vi "Start Wfms.vi"(8 "error in (no error)":errorcluster, 11 "Compiled.Settings":T2={"Name"="", "Async Init Timeout"=0, "File Data"={"Date Captured"="", "Directory"="", "Name"="", "Groups"=[], "Meta Data"=[]}, "Segment Files"=FALSE, "Segment Every"=0.0, "Trigger?"=FALSE, "Segment by"=enum."Size (MB)", "Trigger Ref"=0} {"Trigger Ref" format="%.0x"; "File Data"."Groups"."Channels"."Data Reference in" format="%.0x"}) -> (0 "error out":errorcluster, 1 "Channel Refs":T1[](array[typedef]) format="%.0x", 2 "Wfm Refs":refnum<class "Single Waveform Read (DBL).lvclass">[](array[class]), 3 "Compiled.Settings Out":T2={"Name"="", "Async Init Timeout"=0, "File Data"={"Date Captured"="", "Directory"="", "Name"="", "Groups"=[], "Meta Data"=[]}, "Segment Files"=FALSE, "Segment Every"=0.0, "Trigger?"=FALSE, "Segment by"=enum."Size (MB)", "Trigger Ref"=0} {"Trigger Ref" format="%.0x"; "File Data"."Groups"."Channels"."Data Reference in" format="%.0x"})   [LabVIEW 2023, in "Embedded TDMS Logger Engine.lvlib"]
uses:
  Embedded TDMS Logger Engine.lvlib
  Shared/Compiled.Settings.ctl
  Shared/FileData.ctl
  Shared/GroupData.ctl
  Shared/Meta Data Item.ctl
  Shared/ChannelData.ctl
  <vilib>/NI VeriStand/Custom Device API/Data Reference.ctl
  Shared/SegmentOptions.ctl
  <vilib>/NI VeriStand/Custom Device Waveform API/Single Waveform Read (DBL)/Single Waveform Read (DBL).lvclass
  <vilib>/NI VeriStand/Custom Device Waveform API/Single Waveform Read (DBL)/NI VeriStand - Open Single Waveform Read Session (DBL).vi
  <vilib>/NI VeriStand/Custom Device Waveform API/NI_VS Custom Device Waveform API.lvlib
  Shared/Embedded TDMS Logger Shared.lvlib
  <vilib>/NI VeriStand/Custom Device API/Custom Device API.lvlib
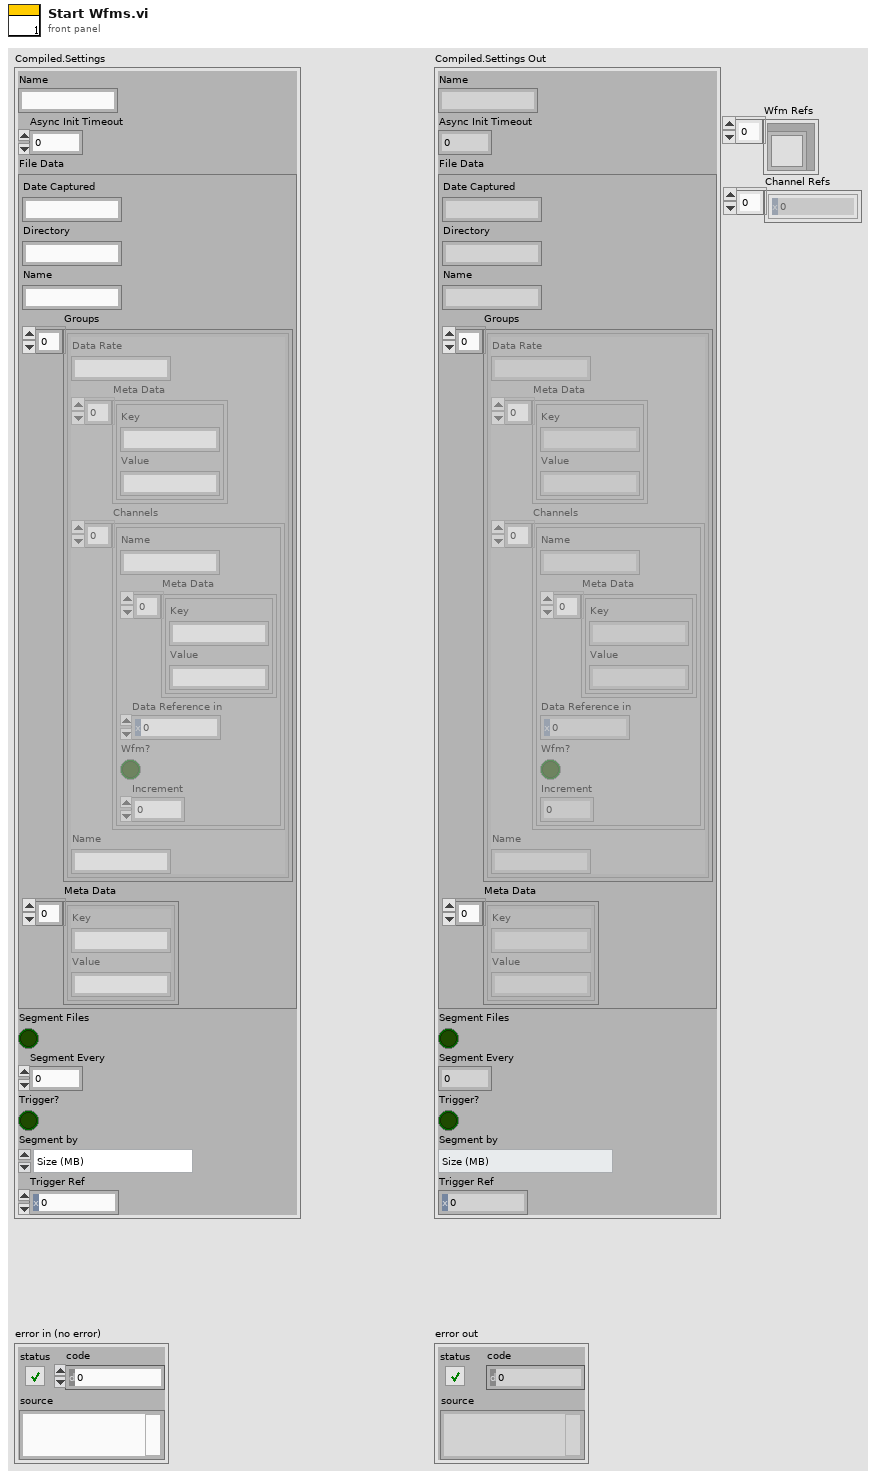
[diagram p1: front panel]
types:
  T1 = typedef "Custom Device API.lvlib/Data Reference.ctl" = i32
  T2 = typedef "Embedded TDMS Logger Shared.lvlib/Compiled.Settings.ctl" = cluster{"Name":string, "Async Init Timeout":u16, "File Data":T3, "Segment Files":bool, "Segment Every":dbl, "Trigger?":bool, "Segment by":T7, "Trigger Ref":T1}
  T3 = typedef "Embedded TDMS Logger Shared.lvlib/FileData.ctl" = cluster{"Date Captured":string, "Directory":string, "Name":string, "Groups":T4[], "Meta Data":T5[]}
  T4 = typedef "Embedded TDMS Logger Shared.lvlib/GroupData.ctl" = cluster{"Data Rate":string, "Meta Data":T5[], "Channels":T6[], "Name":string}
  T5 = typedef "Embedded TDMS Logger Shared.lvlib/Meta Data Item.ctl" = cluster{"Key":string, "Value":string}
  T6 = typedef "Embedded TDMS Logger Shared.lvlib/ChannelData.ctl" = cluster{"Name":string, "Meta Data":T5[], "Data Reference":T1, "Wfm?":bool, "Increment":dbl}
  T7 = typedef "SegmentOptions.ctl" = enum16{"Time (s)", "Size (MB)"}
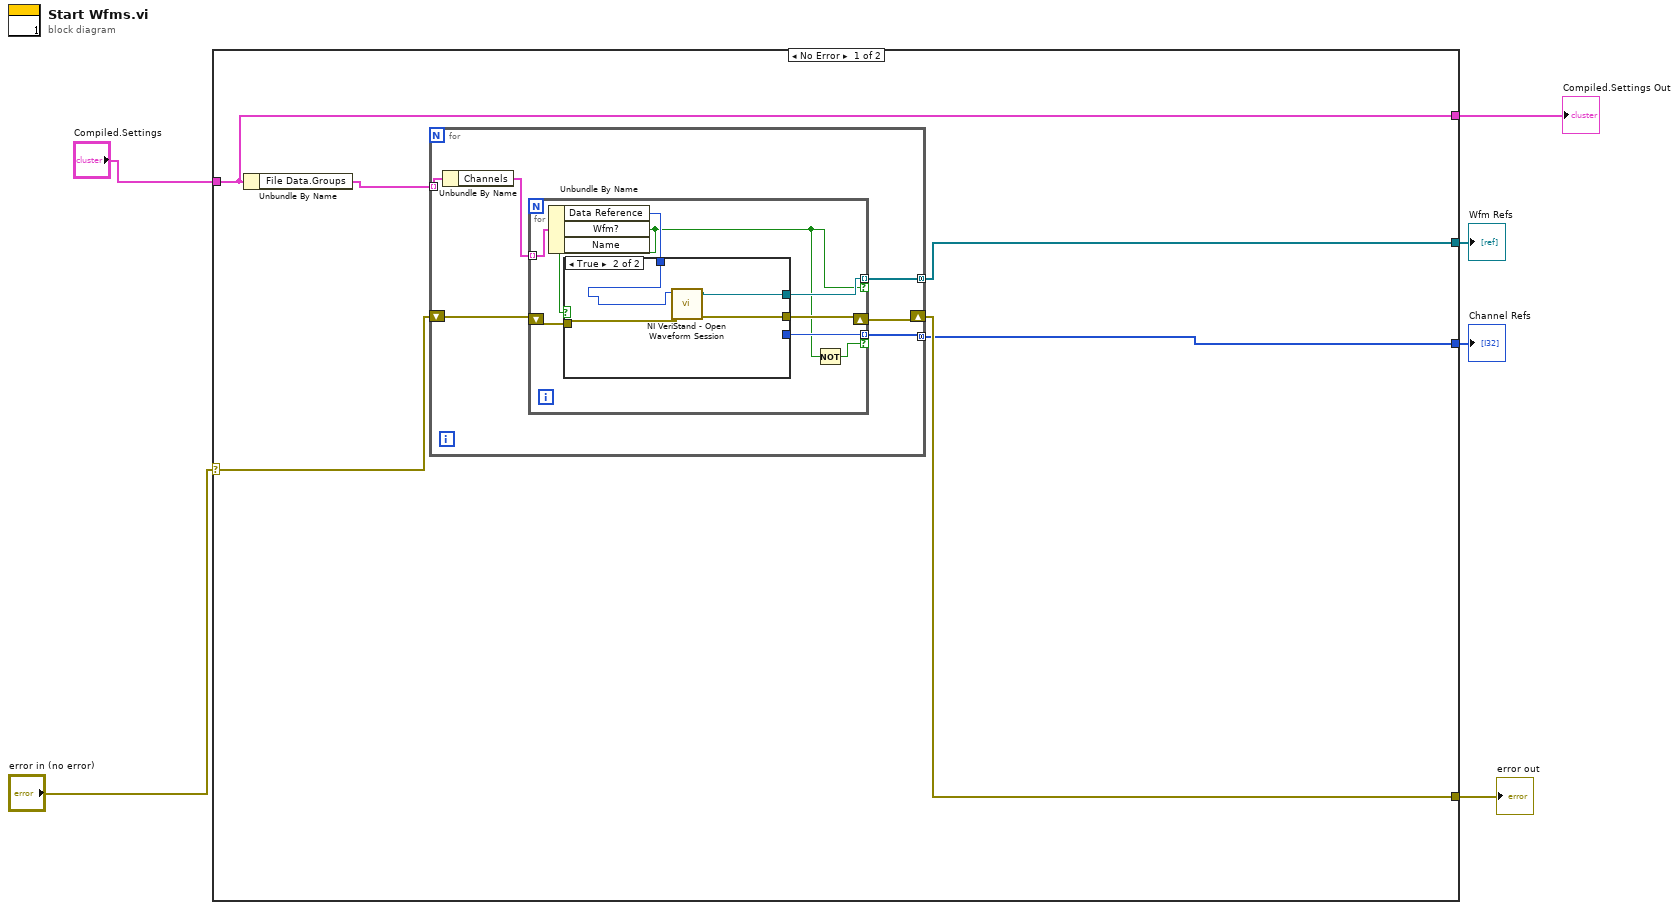
[diagram p0: block diagram]
diagram:
  n1 = case shown="No Error" "error in (no error)" {
    selector: "error in (no error)" -> [w11 w33]
    tunnel: "Compiled.Settings" -> [w9 w34]
    tunnel: [w10 w33] -> w4
    tunnel: [w9 w34] -> w3
    tunnel: [w8 _] -> w2
    tunnel: [w7 _] -> w1
    frame No Error {
      n2 = Unbundle By Name(w9) -> ("File Data.Groups"=w12:T4[])
      n3 = for {
        tunnel: w12 -> [w18] mode=indexing
        shift-right: [w15] -> w10
        shift-left: w11 -> [w16]
        tunnel: [w14] -> w8 mode=concatenating
        tunnel: [w13] -> w7 mode=concatenating
        n4 = Unbundle By Name(w18) -> ("Channels"=w17:T6[])
        n5 = for {
          tunnel: w17 -> [w26] mode=indexing
          shift-right: [w22] -> w15
          shift-left: w16 -> [w24]
          tunnel: [w23] -> w14 mode=indexing if=w19
          tunnel: [w21] -> w13 mode=indexing if=w20
          n6 = Unbundle By Name(w26) -> ("Data Reference"=w25:T1, "Wfm?"=w19:bool)  [unwired: 1 out]
          n7 = case shown="True" w19 {
            tunnel: w25 -> [w28 w30]
            tunnel: w24 -> [w27 w29]
            tunnel: [_ w32] -> w23
            tunnel: [w27 w31] -> w22
            tunnel: [w28 _] -> w21
            frame False {
            }
            frame True {
              n8 = call-poly <vilib>:"NI VeriStand - Open Waveform Session.vi"("error in (no error)"=w29, "DBL Waveform Data Reference"=w30) -> ("error out"=w31:errorcluster, "Single Waveform Read Session (DBL)"=w32:refnum<class "Single Waveform Read (DBL).lvclass">)  [unwired: 8 in]
            }
          }
          n9 = Not(x=w19) -> (.not. x?=w20:bool)
        }
      }
    }
    frame Error {
    }
  }
  "error out" <- w4
  "Compiled.Settings Out" <- w3
  "Wfm Refs" <- w2
  "Channel Refs" <- w1
